vi "List Topic Subscriptions Recursive.vi"(8 "error in (no error)":errorcluster, 10 "NextToken":string, 11 "Topic":refnum<class "Topic.lvclass">) -> (0 "error out":errorcluster, 3 "Topic Subscriptions":refnum<class "Subscription.lvclass">[](array[class]))   [LabVIEW 2015, in "NI_AWS_SNS.lvlib" / "Topic.lvclass"]
uses:
  Topic.lvclass
  Subscription/Subscription.lvclass
  Core/HTTP Request/Request Options.ctl
  Core/HTTP Request/Name Value Pair.ctl
  Core/HTTP Request/Region handling.ctl
  Core/HTTP Request/URL formatting.ctl
  Core/ARN/ARN.lvclass/ARN.ctl
  Core/HTTP Request/HTTP Request.lvclass/HTTP Request.ctl
  Core/ARN/Read ARN.vi
  Core/HTTP Request/Read Credentials.vi
  Core/HTTP Request/Read Service.vi
  Core/HTTP Request/Read Verify Server.vi
  Core/HTTP Request/Write Credentials.vi
  Core/HTTP Request/Write Region.vi
  Core/HTTP Request/Write Service.vi
  Core/HTTP Request/Write Verify Server.vi
  Core/HTTP Request/HTTP Request.lvclass
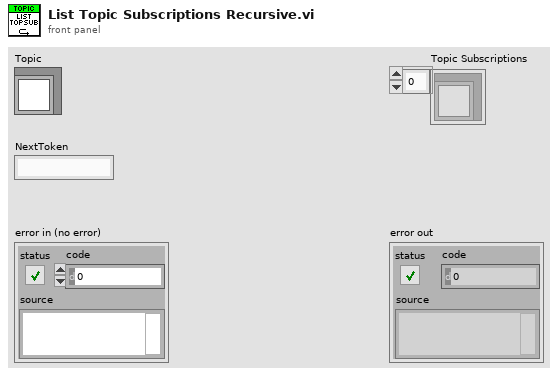
[diagram p1: front panel]
types:
  T1 = typedef "NI_AWS_Core.lvlib/HTTP Request.lvclass/Name Value Pair.ctl" = cluster{"name":string, "value":string}
  T2 = typedef "NI_AWS_Core.lvlib/HTTP Request.lvclass/Request Options.ctl" = cluster{"request headers":T1[], "request parameters":T1[], "request body":string, "region handling":T3, "URL formatting":T4}
  T3 = typedef "NI_AWS_Core.lvlib/HTTP Request.lvclass/Region handling.ctl" = enum16{"use region everywhere", "use region (authentication only)", "use region (URL only)", "ignore region everwhere"}
  T4 = typedef "NI_AWS_Core.lvlib/HTTP Request.lvclass/URL formatting.ctl" = enum16{"region-", "region."}
  T5 = typedef "NI_AWS_Core.lvlib/HTTP Request.lvclass/Response.ctl" = cluster{"Headers":string, "Body":string}
  T6 = typedef "NI_AWS_Core.lvlib/HTTP Request.lvclass/AWS Credentials.ctl" = cluster{"Access Key":string, "Secret Key":string}
  T7 = typedef "NI_AWS_Core.lvlib/HTTP Request.lvclass/Region.ctl" = enum16{"us-east-1", "us-east-2", "us-west-1", "us-west-2", "ap-northeast-1", "ap-northeast-2", "ap-southeast-1", "ap-southeast-2", "ca-central-1", "eu-central-1", "eu-west-1", "eu-west-2", "sa-east-1"}
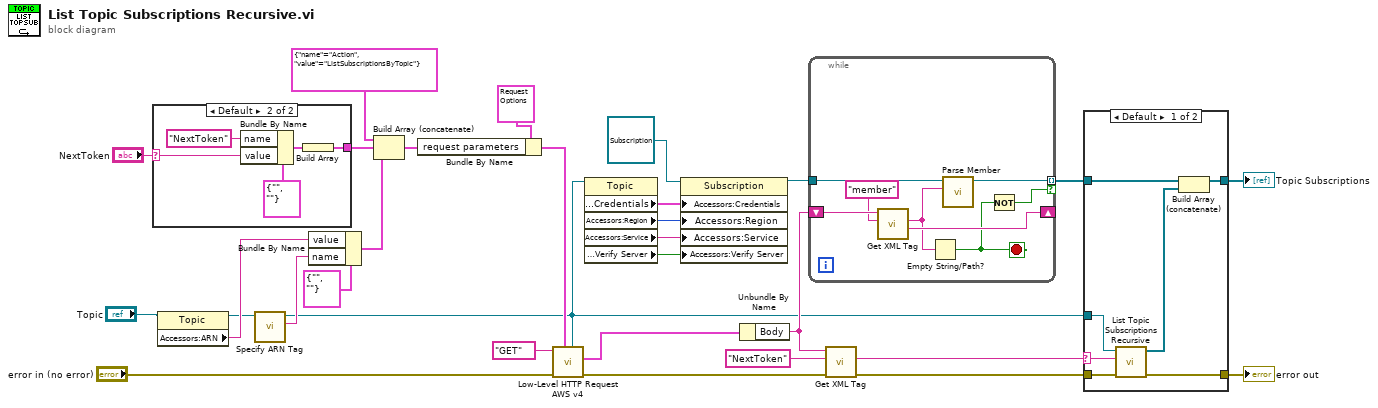
[diagram p0: block diagram]
diagram:
  n1 = case shown="Default" "NextToken" {
    selector: "NextToken" -> [_ w35]
    tunnel: [_ w31] -> w28
    frame "" {
    }
    frame Default {
      n2 = Bundle By Name(cluster=T1 {"name"="", "value"=""} ("Name Value Pair"), "name"="NextToken", "value"=w35) -> (w33:T1)
      n3 = Build Array(w33) -> (w31:T1[])
    }
  }
  n4 = property class="Topic"(reference="Topic") -> (reference out=w13:refnum<class "Topic.lvclass">, "Accessors:ARN"=w14:string)  [unwired: 1 in, 1 out]
  n5 = call-dynamic "Specify ARN Tag.vi"("Topic in"=w13) -> ("ARN Tag"=w10:string, "Topic out"=w1:refnum<class "Topic.lvclass">)  [unwired: 9 in]
  n6 = Bundle By Name(cluster=T1 {"name"="", "value"=""} ("element"), "value"=w14, "name"=w10) -> (w11:T1)
  n7 = Build Array (concatenate)(T1 {"name"="Action", "value"="ListSubscriptionsByTopic"} ("Name Value Pair"), w28, w11) -> (w26:T1[])
  n8 = Bundle By Name(cluster=T2 {"request headers"=[], "request parameters"=[{"name"="Action", "value"="ListQueues"}], "request body"="", "region handling"=enum."use region everywhere", "URL formatting"=enum."region."} ("Request Options"), "request parameters"=w26) -> (w25:T2)
  n9 = call "Low-Level HTTP Request AWS v4.vi"("AWS Core"=w1, "Request Options"=w25, "error in (no error)"="error in (no error)", "HTTP-Verb"="GET") -> ("error out"=w17:errorcluster, "Response"=w30:T5)  [unwired: 5 in, 1 out]
  n10 = property class="Topic"(reference=w1) -> ("Accessors:Credentials"=w5:T6, "Accessors:Region"=w4:T7, "Accessors:Service"=w3:string, "Accessors:Verify Server"=w2:bool)  [unwired: 1 in, 2 out]
  n11 = property class="Subscription"(reference=refnum<class "Subscription.lvclass"> refnum ("NI_AWS_SNS.lvlib:Subscription"), "Accessors:Credentials"=w5, "Accessors:Region"=w4, "Accessors:Service"=w3, "Accessors:Verify Server"=w2) -> (reference out=w6:refnum<class "Subscription.lvclass">)  [unwired: 1 in, 1 out]
  n12 = Unbundle By Name(w30) -> ("Body"=w9:string)
  n13 = while {
    shift-right: [w41] -> _
    shift-left: w9 -> [w43]
    tunnel: [w40] -> w8 mode=indexing if=w37
    tunnel: w6 -> [w36]
    stop <- w38 stop-if-true
    n14 = call "Get XML Tag.vi"("Tag name"="member", "XML String in"=w43) -> ("Remaining string"=w41:string, "Tag value"=w39:string)  [unwired: 5 in, 3 out]
    n15 = Empty String/Path?(string/path=w39) -> (empty?=w38:bool)
    n16 = call-dynamic "Parse Member.vi"("member"=w39, "Subscription in"=w36) -> ("Subscription out"=w40:refnum<class "Subscription.lvclass">)  [unwired: 8 in, 1 out]
    n17 = Not(x=w38) -> (.not. x?=w37:bool)
  }
  n18 = call "Get XML Tag.vi"("error in (no error)"=w17, "Tag name"="NextToken", "XML String in"=w9) -> ("error out"=w16:errorcluster, "Tag value"=w20:string)  [unwired: 4 in, 3 out]
  n19 = case shown="Default" w20 {
    selector: w20 -> [w46 _]
    tunnel: w8 -> [w50 w52]
    tunnel: [w49 w52] -> w19
    tunnel: w16 -> [w48 w51]
    tunnel: [w47 w51] -> w18
    tunnel: w1 -> [w45 _]
    frame Default {
      n20 = call "List Topic Subscriptions Recursive.vi"("error in (no error)"=w48, "NextToken"=w46, "Topic"=w45) -> ("error out"=w47:errorcluster, "Topic Subscriptions"=w44:refnum<class "Subscription.lvclass">[])  [unwired: 7 in]
      n21 = Build Array (concatenate)(w50, w44) -> (w49:refnum<class "Subscription.lvclass">[])
    }
    frame "" {
    }
  }
  "error out" <- w18
  "Topic Subscriptions" <- w19
